vi "Ejercicio 2.3.vi"() -> ()   [LabVIEW 2020]
panel:
  out "Temperatura (°C)":i32
  out "Thermometer":dbl(slide) scale=0.0..100.0
  out "Tanque":i32
  out "Tank":dbl(slide) scale=0.0..12.0
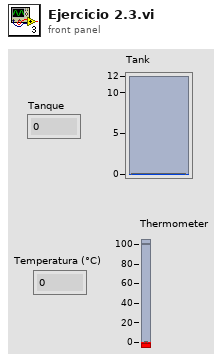
[diagram p1: front panel]
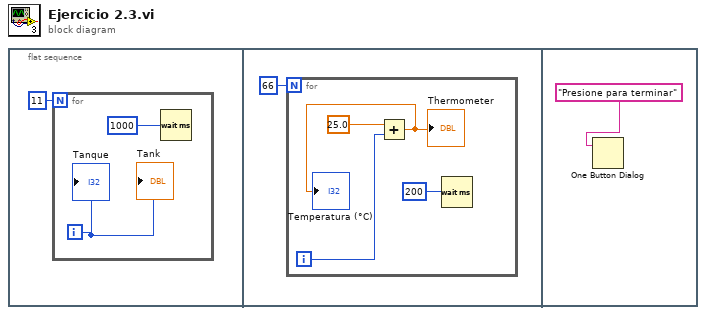
[diagram p0: block diagram]
diagram:
  n1 = flat-sequence {
    frame #0 {
      n2 = for {
        N: 11 -> [_]
        i -> [w2]
        n3 = Wait (ms)(milliseconds to wait=u32 1000) -> ()  [unwired: 1 out]
        "Tank" <- w2
        "Tanque" <- w2
      }
    }
    frame #1 {
      n4 = for {
        N: 66 -> [_]
        i -> [w7]
        n5 = Add(x=25.0 ("Thermometer"), y=w7) -> (x+y=→"Thermometer" →"Temperatura (°C)":dbl)
        n6 = Wait (ms)(milliseconds to wait=u32 200 ("millisecond timer value")) -> ()  [unwired: 1 out]
      }
    }
    frame #2 {
      n7 = One Button Dialog(message="Presione para terminar") -> ()  [unwired: 1 in, 1 out]
    }
  }
